vi "TestSingleMFC.vi"() -> ()   [LabVIEW 2019]
panel:
  out "error out":errorcluster
  in  "Communication Settings":T1={"Unit ID"="A", "Baud Rate"=enum."19200", "VISA Sesssion In"="ASRL13::INSTR"}
  out "MFC_Data":string[](array[string])
  in  "MFC info":T2={"MFC IDs"=["A", "B", "C", "D", "E"], "Setpoint"=[0.0, 0.0, 0.0, 0.0, 0.0], "Max Flow"=[1.0, 1.0, 1.0, 1.0, 1.0]}
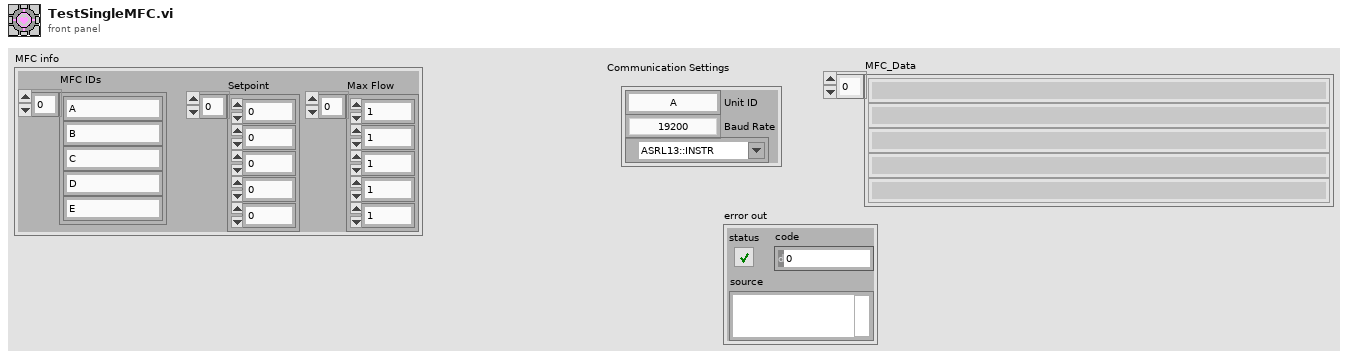
[diagram p1: front panel]
types:
  T1 = cluster{"Unit ID":string, "Baud Rate":enum8{"2400", "9600", "19200", "38400", "57600", "115200", "Unknown"}, "VISA Sesssion In":refnum<visa-resource-name>}
  T2 = cluster{"MFC IDs":string[], "Setpoint":dbl[], "Max Flow":dbl[]}
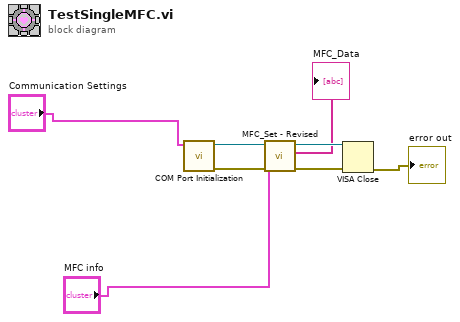
[diagram p0: block diagram]
diagram:
  n1 = call <instrlib>:"COM Port Initialization.vi"("Communication Settings"="Communication Settings") -> ("error out"=w6:errorcluster, "VISA Session Out"=w8:refnum<visa-resource-name>)  [unwired: 9 in]
  n2 = call "MFC_Set - Revised.vi"("error in"=w6, "MFC info"="MFC info", "VISA Session In"=w8) -> ("error out"=w5:errorcluster, "MFC_Data"=→"MFC_Data":string[], "VISA Sesssion Out"=w7:refnum<visa-resource-name>)  [unwired: 6 in]
  n3 = VISA Close(VISA resource name=w7, error in (no error)=w5) -> (error out=→"error out":errorcluster)
